vi "Pontentiometer Check.vi"() -> (2 "Numeric 0":dbl, 3 "Numeric 1":dbl)   [LabVIEW 2015]
uses:
  <vilib>/addons/control/pid/pid.llb/PID (DBL).vi
  <vilib>/addons/control/pid/NI_PID_pid.lvlib
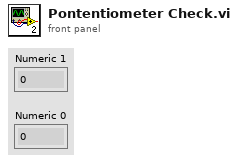
[diagram p1: front panel]
types:
  T1 = typedef "WPI_PotentiometerDevRef.ctl" = cluster{"DevStatus":errorcluster, "Analog Channel":T2, "Invert Output":bool}
  T2 = typedef "FPGA_AIChannel.ctl" = enum8{"AI 0", "AI 1", "AI 2", "AI 3", "AI MXP 0", "AI MXP 1", "AI MXP 2", "AI MXP 3", "Invalid"}
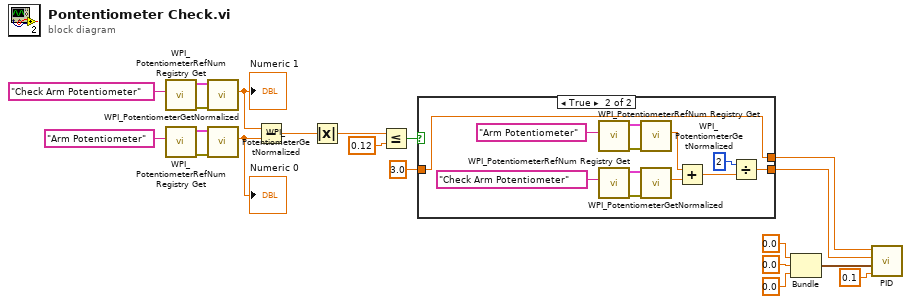
[diagram p0: block diagram]
diagram:
  n1 = call <vilib>:"WPI_PotentiometerRefNum Registry Get.vi"("refnum name"="Check Arm Potentiometer") -> ("error out"=w5:errorcluster, "PotDevRef"=w19:T1)  [unwired: 9 in]
  n2 = call <vilib>:"WPI_PotentiometerRefNum Registry Get.vi"("refnum name"="Arm Potentiometer") -> ("error out"=w6:errorcluster, "PotDevRef"=w17:T1)  [unwired: 9 in]
  n3 = call <vilib>:"WPI_PotentiometerGetNormalized.vi"("error in"=w5, "PotDevRef"=w19) -> ("Normalized Value"=w8:dbl)  [unwired: 7 in, 2 out]
  "Numeric 1" <- w8
  n4 = call <vilib>:"WPI_PotentiometerGetNormalized.vi"("error in"=w6, "PotDevRef"=w17) -> ("Normalized Value"=w7:dbl)  [unwired: 7 in, 2 out]
  "Numeric 0" <- w7
  n5 = Subtract(x=w8, y=w7) -> (x-y=w11:dbl)
  n6 = Absolute Value(x=w11) -> (abs(x)=w10:dbl)
  n7 = Less Or Equal?(x=w10, y=0.12) -> (x <= y?=w3:bool)
  n8 = case shown="True" w3 {
    tunnel: [w21 w23] -> w4
    tunnel: 3.0 -> [w21 w22]
    tunnel: [w21 w22] -> w1
    frame False {
    }
    frame True {
      n9 = call <vilib>:"WPI_PotentiometerRefNum Registry Get.vi"("refnum name"="Arm Potentiometer") -> ("error out"=w32:errorcluster, "PotDevRef"=w33:T1)  [unwired: 9 in]
      n10 = call <vilib>:"WPI_PotentiometerRefNum Registry Get.vi"("refnum name"="Check Arm Potentiometer") -> ("error out"=w30:errorcluster, "PotDevRef"=w31:T1)  [unwired: 9 in]
      n11 = call <vilib>:"WPI_PotentiometerGetNormalized.vi"("error in"=w32, "PotDevRef"=w33) -> ("Normalized Value"=w26:dbl)  [unwired: 7 in, 2 out]
      n12 = call <vilib>:"WPI_PotentiometerGetNormalized.vi"("error in"=w30, "PotDevRef"=w31) -> ("Normalized Value"=w27:dbl)  [unwired: 7 in, 2 out]
      n13 = Add(x=w26, y=w27) -> (x+y=w25:dbl)
      n14 = Divide(x=2, y=w25) -> (x/y=w23:dbl)
    }
  }
  n15 = Bundle(0.0, 0.0, 0.0) -> (w12:cluster{dbl, dbl, dbl})  [unwired: 1 in]
  n16 = call-poly <vilib>:"PID.vi"("dt (s)"=0.1, "PID gains"=w12, "process variable"=w4, "setpoint"=w1) -> ()  [unwired: 6 in, 2 out]
